vi "GetPanesColors.vi"(8 "error in (no error)":errorcluster, 11 "Panes":T2) -> (0 "error out":errorcluster, 3 "Colors":T1)   [LabVIEW 2022 SP3, in "PentaPanesLibrary.lvlib" / "PentaPanes.lvclass"]
uses:
  PentaPanes.lvclass
  PanesCluster.ctl
  PanesColors.ctl
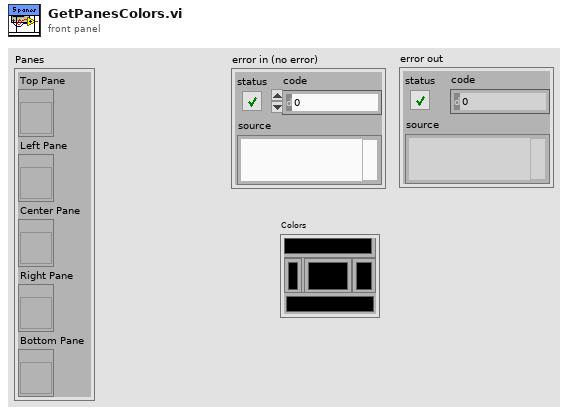
[diagram p1: front panel]
types:
  T1 = typedef "PentaPanesLibrary.lvlib/PentaPanes.lvclass/PanesColors.ctl" = cluster{"Top Color":u32, "Left Color":u32, "Center Color":u32, "Right Color":u32, "Bottom Color":u32}
  T2 = typedef "PentaPanesLibrary.lvlib/PentaPanes.lvclass/PanesCluster.ctl" = cluster{"Top Pane":refnum<vi>, "Left Pane":refnum<vi>, "Center Pane":refnum<vi>, "Right Pane":refnum<vi>, "Bottom Pane":refnum<vi>}
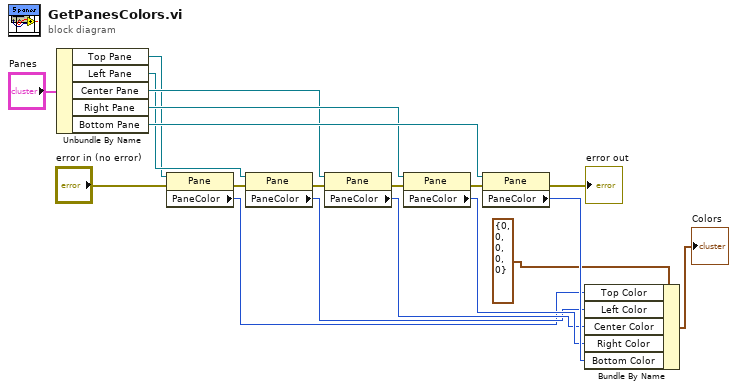
[diagram p0: block diagram]
diagram:
  n1 = Unbundle By Name("Panes") -> ("Top Pane"=w11:refnum<vi>, "Left Pane"=w16:refnum<vi>, "Center Pane"=w17:refnum<vi>, "Right Pane"=w18:refnum<vi>, "Bottom Pane"=w19:refnum<vi>)
  n2 = property class="Pane"(reference=w11, error in="error in (no error)") -> (error out=w9:errorcluster, "PaneColor"=w3:u32)  [unwired: 1 out]
  n3 = property class="Pane"(reference=w16, error in=w9) -> (error out=w8:errorcluster, "PaneColor"=w12:u32)  [unwired: 1 out]
  n4 = property class="Pane"(reference=w17, error in=w8) -> (error out=w7:errorcluster, "PaneColor"=w13:u32)  [unwired: 1 out]
  n5 = property class="Pane"(reference=w18, error in=w7) -> (error out=w6:errorcluster, "PaneColor"=w14:u32)  [unwired: 1 out]
  n6 = property class="Pane"(reference=w19, error in=w6) -> (error out=→"error out":errorcluster, "PaneColor"=w15:u32)  [unwired: 1 out]
  n7 = Bundle By Name(cluster=T1 {"Top Color"=0, "Left Color"=0, "Center Color"=0, "Right Color"=0, "Bottom Color"=0} ("Colors"), "Top Color"=w3, "Left Color"=w12, "Center Color"=w13, "Right Color"=w14, "Bottom Color"=w15) -> (→"Colors":T1)
